vi "Lab Panel V5.28.vi"() -> ()   [LabVIEW 2013] (continued)
                            n1469 = local write "DISP LAB04-1"(w2755) -> ()
                          }
                        }
                      }
                      frame False {
                      }
                    }
                  }
                }
              }
              frame #7 {
                # "LAB04-2"
                n1470 = Equal?(x=w2758, y=2) -> (x = y?=w2761:bool)
                n1471 = local read "DISP LAB04-2"() -> (w2763:T4)
                n1472 = Unbundle(w2763) -> ("STATUS"=w2764:string)  [unwired: 2 out]
                n1473 = Equal?(x=w2764, y="RUN") -> (x = y?=w2760:bool)
                n1474 = And(x=w2760, y=w2761) -> (x .and. y?=w2759:bool)
                n1475 = case shown="True" w2759 {
                  tunnel: w2763 -> [_ w2767]
                  tunnel: w2757 -> [_ w2770]
                  frame False {
                  }
                  frame True {
                    n1476 = local read "SET LAB04-2"() -> (w2769:T5)
                    n1477 = local read "TDMS LAB04-2"() -> (w2766:refnum<k34>)
                    n1478 = Unbundle(w2767) -> ("CYCLE"=w2771:dbl)  [unwired: 2 out]
                    n1479 = Unbundle(w2769) -> ("T-RISE mins"=w2768:dbl)  [unwired: 4 out]
                    n1480 = Greater Or Equal?(x=w2771, y=w2770) -> (x >= y?=w2772:bool)
                    n1481 = case shown="True" w2772 {
                      tunnel: w2768 -> [w2775 _]
                      tunnel: w2767 -> [w2774 _]
                      tunnel: w2766 -> [w2773 _]
                      frame True {
                        n1482 = stacked-sequence {
                          tunnel: w2775 -> [w2778 _]
                          tunnel: w2774 -> [_ w2783]
                          tunnel: w2773 -> [w2776 _]
                          frame #0 {
                            n1483 = Build Array("T-RISE") -> (w2780:string[])
                            n1484 = Build Array(w2778) -> (w2779:dbl[])
                            n1485 = TDMS Write(0:w2776, 5:"TEST PASS", 7:w2780, 9:w2779) -> (15:w2782:errorcluster)  [unwired: 2 in, 3 out]
                            n1486 = local write "data file error"(w2782) -> ()
                          }
                          frame #1 {
                            n1487 = Bundle(cluster=w2783, "STATUS"="T-RISE PASS") -> (w2785:T4)  [unwired: 2 in]
                            n1488 = local write "RESULT LAB04-2"(TRUE) -> ()
                            n1489 = local write "DISP LAB04-2"(w2785) -> ()
                          }
                        }
                      }
                      frame False {
                      }
                    }
                  }
                }
              }
              frame #8 {
                # "LAB05-1"
                n1490 = Equal?(x=w2788, y=2) -> (x = y?=w2791:bool)
                n1491 = local read "DISP LAB05-1"() -> (w2793:T4)
                n1492 = Unbundle(w2793) -> ("STATUS"=w2794:string)  [unwired: 2 out]
                n1493 = Equal?(x=w2794, y="RUN") -> (x = y?=w2790:bool)
                n1494 = And(x=w2790, y=w2791) -> (x .and. y?=w2789:bool)
                n1495 = case shown="True" w2789 {
                  tunnel: w2793 -> [_ w2797]
                  tunnel: w2787 -> [_ w2800]
                  frame False {
                  }
                  frame True {
                    n1496 = local read "SET LAB05-1"() -> (w2799:T5)
                    n1497 = local read "TDMS LAB05-1"() -> (w2796:refnum<k34>)
                    n1498 = Unbundle(w2797) -> ("CYCLE"=w2801:dbl)  [unwired: 2 out]
                    n1499 = Unbundle(w2799) -> ("T-RISE mins"=w2798:dbl)  [unwired: 4 out]
                    n1500 = Greater Or Equal?(x=w2801, y=w2800) -> (x >= y?=w2802:bool)
                    n1501 = case shown="True" w2802 {
                      tunnel: w2798 -> [w2805 _]
                      tunnel: w2797 -> [w2804 _]
                      tunnel: w2796 -> [w2803 _]
                      frame True {
                        n1502 = stacked-sequence {
                          tunnel: w2805 -> [w2808 _]
                          tunnel: w2804 -> [_ w2813]
                          tunnel: w2803 -> [w2806 _]
                          frame #0 {
                            n1503 = Build Array("T-RISE") -> (w2810:string[])
                            n1504 = Build Array(w2808) -> (w2809:dbl[])
                            n1505 = TDMS Write(0:w2806, 5:"TEST PASS", 7:w2810, 9:w2809) -> (15:w2812:errorcluster)  [unwired: 2 in, 3 out]
                            n1506 = local write "data file error"(w2812) -> ()
                          }
                          frame #1 {
                            n1507 = Bundle(cluster=w2813, "STATUS"="T-RISE PASS") -> (w2815:T4)  [unwired: 2 in]
                            n1508 = local write "RESULT LAB05-1"(TRUE) -> ()
                            n1509 = local write "DISP LAB05-1"(w2815) -> ()
                          }
                        }
                      }
                      frame False {
                      }
                    }
                  }
                }
              }
              frame #9 {
                # "LAB05-2"
                n1510 = Equal?(x=w2818, y=2) -> (x = y?=w2821:bool)
                n1511 = local read "DISP LAB05-2"() -> (w2823:T4)
                n1512 = Unbundle(w2823) -> ("STATUS"=w2824:string)  [unwired: 2 out]
                n1513 = Equal?(x=w2824, y="RUN") -> (x = y?=w2820:bool)
                n1514 = And(x=w2820, y=w2821) -> (x .and. y?=w2819:bool)
                n1515 = case shown="True" w2819 {
                  tunnel: w2823 -> [_ w2827]
                  tunnel: w2817 -> [_ w2830]
                  frame False {
                  }
                  frame True {
                    n1516 = local read "SET LAB05-2"() -> (w2829:T5)
                    n1517 = local read "TDMS LAB05-2"() -> (w2826:refnum<k34>)
                    n1518 = Unbundle(w2827) -> ("CYCLE"=w2831:dbl)  [unwired: 2 out]
                    n1519 = Unbundle(w2829) -> ("T-RISE mins"=w2828:dbl)  [unwired: 4 out]
                    n1520 = Greater Or Equal?(x=w2831, y=w2830) -> (x >= y?=w2832:bool)
                    n1521 = case shown="True" w2832 {
                      tunnel: w2828 -> [w2835 _]
                      tunnel: w2827 -> [w2834 _]
                      tunnel: w2826 -> [w2833 _]
                      frame True {
                        n1522 = stacked-sequence {
                          tunnel: w2835 -> [w2838 _]
                          tunnel: w2834 -> [_ w2843]
                          tunnel: w2833 -> [w2836 _]
                          frame #0 {
                            n1523 = Build Array("T-RISE") -> (w2840:string[])
                            n1524 = Build Array(w2838) -> (w2839:dbl[])
                            n1525 = TDMS Write(0:w2836, 5:"TEST PASS", 7:w2840, 9:w2839) -> (15:w2842:errorcluster)  [unwired: 2 in, 3 out]
                            n1526 = local write "data file error"(w2842) -> ()
                          }
                          frame #1 {
                            n1527 = Bundle(cluster=w2843, "STATUS"="T-RISE PASS") -> (w2845:T4)  [unwired: 2 in]
                            n1528 = local write "RESULT LAB05-2"(TRUE) -> ()
                            n1529 = local write "DISP LAB05-2"(w2845) -> ()
                          }
                        }
                      }
                      frame False {
                      }
                    }
                  }
                }
              }
            }
          }
          frame #7 {
            # "end test & close test files"
            n1530 = local read "MAIL SETTINGS"() -> (w2852:T7)
            n1531 = local read "TO (string):"() -> (w2847:string)
            n1532 = Unbundle(w2852) -> ("OUT SERVER ADDRESS"=w2851:string, "FROM ACCOUNT"=w2850:string)  [unwired: 5 out]
            n1533 = stacked-sequence {
              tunnel: w2862 -> [_ _ _ _ _ _ _ _ _ _]
              tunnel: w2863 -> [_ _ _ _ _ _ _ _ _ _]
              tunnel: w2861 -> [_ _ _ _ _ _ _ _ _ _]
              tunnel: w2860 -> [_ _ _ _ _ _ _ _ _ _]
              tunnel: w2859 -> [_ _ _ _ _ _ _ _ _ _]
              tunnel: w2858 -> [_ _ _ _ _ _ _ _ _ _]
              tunnel: w2857 -> [_ _ _ _ _ _ _ _ _ _]
              tunnel: w2856 -> [_ _ _ _ _ _ _ _ _ _]
              tunnel: w2855 -> [_ _ _ _ _ _ _ _ _ _]
              tunnel: w2854 -> [_ _ _ _ _ _ _ _ _ _]
              tunnel: w2851 -> [w2868 w2919 w2967 w3014 w3061 w3108 w3155 w3202 w3249 w3296]
              tunnel: w2850 -> [w2867 w2918 w2966 w3013 w3060 w3107 w3154 w3201 w3248 w3295]
              tunnel: "Mail Test File To:" -> [w2866 w2917 w2965 w3012 w3059 w3106 w3153 w3200 w3247 w3294]
              tunnel: "Mail Test Fail" -> [w2865 w2916 w2964 w3011 w3058 w3105 w3152 w3199 w3246 w3293]
              frame #0 {
                # "LAB01-1"
                n1534 = local read "DISP LAB01-1"() -> (w2864:T4)
                n1535 = global write "Global display 2.vi" "DISP LAB01-1"(w2864) -> ()
                n1536 = local read "run lab01-1"() -> (w2869:bool)
                n1537 = local read "TDMS LAB01-1"() -> (w2870:refnum<k34>)
                n1538 = Unbundle(w2864) -> ("CYCLE"=w2872:dbl, "STATUS"=w2871:string)  [unwired: 1 out]
                n1539 = case shown="True" w2869 {
                  tunnel: w2872 -> [_ w2878]
                  tunnel: w2864 -> [_ w2880]
                  tunnel: w2871 -> [_ w2877]
                  tunnel: w2870 -> [_ w2879]
                  tunnel: w2868 -> [_ w2876]
                  tunnel: w2867 -> [_ w2875]
                  tunnel: w2866 -> [_ w2874]
                  tunnel: w2865 -> [_ w2873]
                  frame False {
                  }
                  frame True {
                    n1540 = Not Equal?(x=w2877, y="RUN") -> (x != y?=w2881:bool)
                    n1541 = Greater?(x=w2878, y=2.0) -> (0:w2883:bool)
                    n1542 = And(x=w2883, y=w2881) -> (x .and. y?=w2882:bool)
                    n1543 = case shown="True" w2882 {
                      tunnel: w2880 -> [_ w2893]
                      tunnel: w2879 -> [_ w2892]
                      tunnel: w2878 -> [_ w2891]
                      tunnel: w2877 -> [_ w2890]
                      tunnel: w2876 -> [_ w2889]
                      tunnel: w2875 -> [_ w2888]
                      tunnel: w2874 -> [_ w2887]
                      tunnel: w2873 -> [_ w2886]
                      frame False {
                      }
                      frame True {
                        n1544 = stacked-sequence {
                          tunnel: w2893 -> [w2897 _ _]
                          tunnel: w2892 -> [_ w2899 _]
                          tunnel: w2891 -> [_ _ _]
                          tunnel: w2890 -> [_ _ w2905]
                          tunnel: w2889 -> [_ _ w2904]
                          tunnel: w2888 -> [_ _ w2903]
                          tunnel: w2887 -> [_ _ w2902]
                          tunnel: w2886 -> [_ _ w2901]
                          frame #0 {
                            w2894 = FALSE
                            n1545 = local write "mail control"("END") -> ()
                            n1546 = Bundle(cluster=w2897) -> (w2896:T4)  [unwired: 3 in]
                            n1547 = local write "DISP LAB01-1"(w2896) -> ()
                            n1548 = local write "O/I  LAB01-1"(w2894) -> ()
                            n1549 = local write "run lab01-1"(w2894) -> ()
                            n1550 = local write "RUN LAB01-1"(w2894) -> ()
                          }
                          frame #1 {
                            n1551 = TDMS Close(11:w2899) -> (0:w2898:errorcluster)  [unwired: 1 in, 1 out]
                            n1552 = local write "data file error"(w2898) -> ()
                          }
                          frame #2 {
                            n1553 = stacked-sequence {
                              tunnel: "LAB01-1" -> [w2907 w2909 _]
                              tunnel: w2905 -> [_ w2915 _]
                              tunnel: w2904 -> [_ w2914 _]
                              tunnel: w2903 -> [_ w2913 _]
                              tunnel: w2902 -> [_ w2912 _]
                              tunnel: w2901 -> [_ w2911 _]
                              frame #0 {
                                n1554 = call "sub vi - defrag tdms v1.vi"("panel id"=w2907) -> ("error out"=w2906:errorcluster)  [unwired: 10 in]
                                n1555 = local write "data file error"(w2906) -> ()
                              }
                              frame #1 {
                                n1556 = Bundle("STATUS"=w2915, "OUT SERVER ADDRESS"=w2914, "FROM ACCOUNT"=w2913, "Mail Test File To:"=w2912, "Mail Test Fail"=w2911) -> (w2908:T26)  [unwired: 1 in]
                                n1557 = call "Save data file (pass-fail) v5.vi"("Input Cluster"=w2908, "panel id"=w2909) -> ("network file save error"=w2910:errorcluster)  [unwired: 8 in, 1 out]
                                n1558 = local write "data file error"(w2910) -> ()
                              }
                              frame #2 {
                              }
                            }
                          }
                        }
                      }
                    }
                  }
                }
              }
              frame #1 {
                # "LAB01-2"
                n1559 = local read "run lab01-2"() -> (w2920:bool)
                n1560 = case shown="True" w2920 {
                  tunnel: w2919 -> [_ w2925]
                  tunnel: w2918 -> [_ w2924]
                  tunnel: w2917 -> [_ w2923]
                  tunnel: w2916 -> [_ w2922]
                  frame False {
                  }
                  frame True {
                    n1561 = local read "DISP LAB01-2"() -> (w2921:T4)
                    n1562 = global write "Global display 2.vi" "DISP LAB01-2"(w2921) -> ()
                    n1563 = local read "TDMS LAB01-2"() -> (w2932:refnum<k34>)
                    n1564 = Unbundle(w2921) -> ("CYCLE"=w2927:dbl, "STATUS"=w2926:string)  [unwired: 1 out]
                    n1565 = Not Equal?(x=w2926, y="RUN") -> (x != y?=w2929:bool)
                    n1566 = Greater?(x=w2927, y=2.0) -> (0:w2930:bool)
                    n1567 = And(x=w2930, y=w2929) -> (x .and. y?=w2928:bool)
                    n1568 = case shown="True" w2928 {
                      tunnel: w2921 -> [_ w2941]
                      tunnel: w2932 -> [_ w2940]
                      tunnel: w2927 -> [_ w2939]
                      tunnel: w2926 -> [_ w2938]
                      tunnel: w2925 -> [_ w2937]
                      tunnel: w2924 -> [_ w2936]
                      tunnel: w2923 -> [_ w2935]
                      tunnel: w2922 -> [_ w2934]
                      frame False {
                      }
                      frame True {
                        n1569 = stacked-sequence {
                          tunnel: w2941 -> [w2944 _ _]
                          tunnel: w2940 -> [_ w2946 _]
                          tunnel: w2939 -> [_ _ _]
                          tunnel: w2938 -> [_ _ w2952]
                          tunnel: w2937 -> [_ _ w2951]
                          tunnel: w2936 -> [_ _ w2950]
                          tunnel: w2935 -> [_ _ w2949]
                          tunnel: w2934 -> [_ _ w2948]
                          frame #0 {
                            w2942 = FALSE
                            n1570 = local write "mail control"("END") -> ()
                            n1571 = Bundle(cluster=w2944) -> (w2945:T4)  [unwired: 3 in]
                            n1572 = local write "RUN LAB01-2"(w2942) -> ()
                            n1573 = local write "run lab01-2"(w2942) -> ()
                            n1574 = local write "O/I  LAB01-2"(w2942) -> ()
                            n1575 = local write "DISP LAB01-2"(w2945) -> ()
                          }
                          frame #1 {
                            n1576 = TDMS Close(11:w2946) -> (0:w2947:errorcluster)  [unwired: 1 in, 1 out]
                            n1577 = local write "data file error"(w2947) -> ()
                          }
                          frame #2 {
                            n1578 = stacked-sequence {
                              tunnel: "LAB01-2" -> [w2955 w2956]
                              tunnel: w2952 -> [_ w2961]
                              tunnel: w2951 -> [_ w2960]
                              tunnel: w2950 -> [_ w2959]
                              tunnel: w2949 -> [_ w2958]
                              tunnel: w2948 -> [_ w2957]
                              frame #0 {
                                n1579 = call "sub vi - defrag tdms v1.vi"("panel id"=w2955) -> ("error out"=w2954:errorcluster)  [unwired: 10 in]
                                n1580 = local write "data file error"(w2954) -> ()
                              }
                              frame #1 {
                                n1581 = Bundle("STATUS"=w2961, "OUT SERVER ADDRESS"=w2960, "FROM ACCOUNT"=w2959, "Mail Test File To:"=w2958, "Mail Test Fail"=w2957) -> (w2963:T26)  [unwired: 1 in]
                                n1582 = call "Save data file (pass-fail) v5.vi"("Input Cluster"=w2963, "panel id"=w2956) -> ("network file save error"=w2962:errorcluster)  [unwired: 8 in, 1 out]
                                n1583 = local write "data file error"(w2962) -> ()
                              }
                            }
                          }
                        }
                      }
                    }
                  }
                }
              }
              frame #2 {
                # "LAB02-1"
                n1584 = local read "run lab02-1"() -> (w2968:bool)
                n1585 = case shown="True" w2968 {
                  tunnel: w2967 -> [_ w2973]
                  tunnel: w2966 -> [_ w2972]
                  tunnel: w2965 -> [_ w2971]
                  tunnel: w2964 -> [_ w2970]
                  frame False {
                  }
                  frame True {
                    n1586 = local read "DISP LAB02-1"() -> (w2969:T4)
                    n1587 = global write "Global display 2.vi" "DISP LAB02-1"(w2969) -> ()
                    n1588 = Unbundle(w2969) -> ("CYCLE"=w2977:dbl, "STATUS"=w2974:string)  [unwired: 1 out]
                    n1589 = local read "TDMS LAB02-1"() -> (w2980:refnum<k34>)
                    n1590 = Not Equal?(x=w2974, y="RUN") -> (x != y?=w2976:bool)
                    n1591 = Greater?(x=w2977, y=2.0) -> (0:w2978:bool)
                    n1592 = And(x=w2978, y=w2976) -> (x .and. y?=w2975:bool)
                    n1593 = case shown="True" w2975 {
                      tunnel: w2969 -> [_ w2988]
                      tunnel: w2980 -> [_ w2987]
                      tunnel: w2974 -> [_ w2986]
                      tunnel: w2973 -> [_ w2985]
                      tunnel: w2972 -> [_ w2984]
                      tunnel: w2971 -> [_ w2983]
                      tunnel: w2970 -> [_ w2982]
                      frame False {
                      }
                      frame True {
                        n1594 = stacked-sequence {
                          tunnel: w2988 -> [w2991 _ _]
                          tunnel: w2987 -> [_ w2993 _]
                          tunnel: w2986 -> [_ _ w2999]
                          tunnel: w2985 -> [_ _ w2998]
                          tunnel: w2984 -> [_ _ w2997]
                          tunnel: w2983 -> [_ _ w2996]
                          tunnel: w2982 -> [_ _ w2995]
                          frame #0 {
                            w2989 = FALSE
                            n1595 = local write "mail control"("END") -> ()
                            n1596 = Bundle(cluster=w2991) -> (w2992:T4)  [unwired: 3 in]
                            n1597 = local write "O/I  LAB02-1"(w2989) -> ()
                            n1598 = local write "RUN LAB02-1"(w2989) -> ()
                            n1599 = local write "run lab02-1"(w2989) -> ()
                            n1600 = local write "DISP LAB02-1"(w2992) -> ()
                          }
                          frame #1 {
                            n1601 = TDMS Close(11:w2993) -> (0:w2994:errorcluster)  [unwired: 1 in, 1 out]
                            n1602 = local write "data file error"(w2994) -> ()
                          }
                          frame #2 {
                            n1603 = stacked-sequence {
                              tunnel: "LAB02-1" -> [w3002 w3009]
                              tunnel: w2999 -> [_ w3007]
                              tunnel: w2998 -> [_ w3006]
                              tunnel: w2997 -> [_ w3005]
                              tunnel: w2996 -> [_ w3004]
                              tunnel: w2995 -> [_ w3003]
                              frame #0 {
                                n1604 = call "sub vi - defrag tdms v1.vi"("panel id"=w3002) -> ("error out"=w3001:errorcluster)  [unwired: 10 in]
                                n1605 = local write "data file error"(w3001) -> ()
                              }
                              frame #1 {
                                n1606 = Bundle("STATUS"=w3007, "OUT SERVER ADDRESS"=w3006, "FROM ACCOUNT"=w3005, "Mail Test File To:"=w3004, "Mail Test Fail"=w3003) -> (w3008:T26)  [unwired: 1 in]
                                n1607 = call "Save data file (pass-fail) v5.vi"("Input Cluster"=w3008, "panel id"=w3009) -> ("network file save error"=w3010:errorcluster)  [unwired: 8 in, 1 out]
                                n1608 = local write "data file error"(w3010) -> ()
                              }
                            }
                          }
                        }
                      }
                    }
                  }
                }
              }
              frame #3 {
                # "LAB02-2"
                n1609 = local read "run lab02-2"() -> (w3015:bool)
                n1610 = case shown="True" w3015 {
                  tunnel: w3014 -> [_ w3021]
                  tunnel: w3013 -> [_ w3020]
                  tunnel: w3012 -> [_ w3019]
                  tunnel: w3011 -> [_ w3018]
                  frame False {
                  }
                  frame True {
                    n1611 = local read "DISP LAB02-2"() -> (w3017:T4)
                    n1612 = global write "Global display 2.vi" "DISP LAB02-2"(w3017) -> ()
                    n1613 = local read "TDMS LAB02-2"() -> (w3027:refnum<k34>)
                    n1614 = Unbundle(w3017) -> ("CYCLE"=w3016:dbl, "STATUS"=w3022:string)  [unwired: 1 out]
                    n1615 = Not Equal?(x=w3022, y="RUN") -> (x != y?=w3024:bool)
                    n1616 = Greater?(x=w3016, y=2.0) -> (0:w3025:bool)
                    n1617 = And(x=w3025, y=w3024) -> (x .and. y?=w3023:bool)
                    n1618 = case shown="True" w3023 {
                      tunnel: w3017 -> [_ w3035]
                      tunnel: w3027 -> [_ w3034]
                      tunnel: w3022 -> [_ w3033]
                      tunnel: w3021 -> [_ w3032]
                      tunnel: w3020 -> [_ w3031]
                      tunnel: w3019 -> [_ w3030]
                      tunnel: w3018 -> [_ w3029]
                      frame False {
                      }
                      frame True {
                        n1619 = stacked-sequence {
                          tunnel: w3035 -> [w3038 _ _]
                          tunnel: w3034 -> [_ w3040 _]
                          tunnel: w3033 -> [_ _ w3046]
                          tunnel: w3032 -> [_ _ w3045]
                          tunnel: w3031 -> [_ _ w3044]
                          tunnel: w3030 -> [_ _ w3043]
                          tunnel: w3029 -> [_ _ w3042]
                          frame #0 {
                            w3036 = FALSE
                            n1620 = local write "mail control"("END") -> ()
                            n1621 = Bundle(cluster=w3038) -> (w3039:T4)  [unwired: 3 in]
                            n1622 = local write "O/I  LAB02-2"(w3036) -> ()
                            n1623 = local write "run lab02-2"(w3036) -> ()
                            n1624 = local write "RUN LAB02-2"(w3036) -> ()
                            n1625 = local write "DISP LAB02-2"(w3039) -> ()
                          }
                          frame #1 {
                            n1626 = TDMS Close(11:w3040) -> (0:w3041:errorcluster)  [unwired: 1 in, 1 out]
                            n1627 = local write "data file error"(w3041) -> ()
                          }
                          frame #2 {
                            n1628 = stacked-sequence {
                              tunnel: "LAB02-2" -> [w3049 w3055]
                              tunnel: w3046 -> [_ w3054]
                              tunnel: w3045 -> [_ w3053]
                              tunnel: w3044 -> [_ w3052]
                              tunnel: w3043 -> [_ w3051]
                              tunnel: w3042 -> [_ w3050]
                              frame #0 {
                                n1629 = call "sub vi - defrag tdms v1.vi"("panel id"=w3049) -> ("error out"=w3048:errorcluster)  [unwired: 10 in]
                                n1630 = local write "data file error"(w3048) -> ()
                              }
                              frame #1 {
                                n1631 = Bundle("STATUS"=w3054, "OUT SERVER ADDRESS"=w3053, "FROM ACCOUNT"=w3052, "Mail Test File To:"=w3051, "Mail Test Fail"=w3050) -> (w3057:T26)  [unwired: 1 in]
                                n1632 = call "Save data file (pass-fail) v5.vi"("Input Cluster"=w3057, "panel id"=w3055) -> ("network file save error"=w3056:errorcluster)  [unwired: 8 in, 1 out]
                                n1633 = local write "data file error"(w3056) -> ()
                              }
                            }
                          }
                        }
                      }
                    }
                  }
                }
              }
              frame #4 {
                # "LAB03-1"
                n1634 = local read "run lab03-1"() -> (w3062:bool)
                n1635 = case shown="True" w3062 {
                  tunnel: w3061 -> [_ w3067]
                  tunnel: w3060 -> [_ w3066]
                  tunnel: w3059 -> [_ w3065]
                  tunnel: w3058 -> [_ w3064]
                  frame False {
                  }
                  frame True {
                    n1636 = local read "DISP LAB03-1"() -> (w3063:T4)
                    n1637 = local read "TDMS LAB03-1"() -> (w3074:refnum<k34>)
                    n1638 = global write "Global display 2.vi" "DISP LAB03-1"(w3063) -> ()
                    n1639 = Unbundle(w3063) -> ("CYCLE"=w3071:dbl, "STATUS"=w3068:string)  [unwired: 1 out]
                    n1640 = Not Equal?(x=w3068, y="RUN") -> (x != y?=w3070:bool)
                    n1641 = Greater?(x=w3071, y=2.0) -> (0:w3072:bool)
                    n1642 = And(x=w3072, y=w3070) -> (x .and. y?=w3069:bool)
                    n1643 = case shown="True" w3069 {
                      tunnel: w3063 -> [_ w3082]
                      tunnel: w3074 -> [_ w3081]
                      tunnel: w3068 -> [_ w3080]
                      tunnel: w3067 -> [_ w3079]
                      tunnel: w3066 -> [_ w3078]
                      tunnel: w3065 -> [_ w3077]
                      tunnel: w3064 -> [_ w3076]
                      frame False {
                      }
                      frame True {
                        n1644 = stacked-sequence {
                          tunnel: w3082 -> [w3085 _ _]
                          tunnel: w3081 -> [_ w3087 _]
                          tunnel: w3080 -> [_ _ w3093]
                          tunnel: w3079 -> [_ _ w3092]
                          tunnel: w3078 -> [_ _ w3091]
                          tunnel: w3077 -> [_ _ w3090]
                          tunnel: w3076 -> [_ _ w3089]
                          frame #0 {
                            w3083 = FALSE
                            n1645 = local write "mail control"("END") -> ()
                            n1646 = Bundle(cluster=w3085) -> (w3086:T4)  [unwired: 3 in]
                            n1647 = local write "O/I  LAB03-1"(w3083) -> ()
                            n1648 = local write "run lab03-1"(w3083) -> ()
                            n1649 = local write "RUN LAB03-1"(w3083) -> ()
                            n1650 = local write "DISP LAB03-1"(w3086) -> ()
                          }
                          frame #1 {
                            n1651 = TDMS Close(11:w3087) -> (0:w3088:errorcluster)  [unwired: 1 in, 1 out]
                            n1652 = local write "data file error"(w3088) -> ()
                          }
                          frame #2 {
                            n1653 = stacked-sequence {
                              tunnel: "LAB03-1" -> [w3096 w3102]
                              tunnel: w3093 -> [_ w3101]
                              tunnel: w3092 -> [_ w3100]
                              tunnel: w3091 -> [_ w3099]
                              tunnel: w3090 -> [_ w3098]
                              tunnel: w3089 -> [_ w3097]
                              frame #0 {
                                n1654 = call "sub vi - defrag tdms v1.vi"("panel id"=w3096) -> ("error out"=w3095:errorcluster)  [unwired: 10 in]
                                n1655 = local write "data file error"(w3095) -> ()
                              }
                              frame #1 {
                                n1656 = Bundle("STATUS"=w3101, "OUT SERVER ADDRESS"=w3100, "FROM ACCOUNT"=w3099, "Mail Test File To:"=w3098, "Mail Test Fail"=w3097) -> (w3104:T26)  [unwired: 1 in]
                                n1657 = call "Save data file (pass-fail) v5.vi"("Input Cluster"=w3104, "panel id"=w3102) -> ("network file save error"=w3103:errorcluster)  [unwired: 8 in, 1 out]
                                n1658 = local write "data file error"(w3103) -> ()
                              }
                            }
                          }
                        }
                      }
                    }
                  }
                }
              }
              frame #5 {
                # "LAB03-2"
                n1659 = local read "run lab03-2"() -> (w3109:bool)
                n1660 = case shown="True" w3109 {
                  tunnel: w3108 -> [_ w3114]
                  tunnel: w3107 -> [_ w3113]
                  tunnel: w3106 -> [_ w3112]
                  tunnel: w3105 -> [_ w3111]
                  frame False {
                  }
                  frame True {
                    n1661 = local read "DISP LAB03-2"() -> (w3110:T4)
                    n1662 = global write "Global display 2.vi" "DISP LAB03-2"(w3110) -> ()
                    n1663 = Unbundle(w3110) -> ("CYCLE"=w3118:dbl, "STATUS"=w3115:string)  [unwired: 1 out]
                    n1664 = local read "TDMS LAB03-2"() -> (w3121:refnum<k34>)
                    n1665 = Not Equal?(x=w3115, y="RUN") -> (x != y?=w3117:bool)
                    n1666 = Greater?(x=w3118, y=2.0) -> (0:w3119:bool)
                    n1667 = And(x=w3119, y=w3117) -> (x .and. y?=w3116:bool)
                    n1668 = case shown="True" w3116 {
                      tunnel: w3110 -> [_ w3129]
                      tunnel: w3121 -> [_ w3128]
                      tunnel: w3115 -> [_ w3127]
                      tunnel: w3114 -> [_ w3126]
                      tunnel: w3113 -> [_ w3125]
                      tunnel: w3112 -> [_ w3124]
                      tunnel: w3111 -> [_ w3123]
                      frame False {
                      }
                      frame True {
                        n1669 = stacked-sequence {
                          tunnel: w3129 -> [w3132 _ _]
                          tunnel: w3128 -> [_ w3134 _]
                          tunnel: w3127 -> [_ _ w3140]
                          tunnel: w3126 -> [_ _ w3139]
                          tunnel: w3125 -> [_ _ w3138]
                          tunnel: w3124 -> [_ _ w3137]
                          tunnel: w3123 -> [_ _ w3136]
                          frame #0 {
                            w3130 = FALSE
                            n1670 = local write "mail control"("END") -> ()
                            n1671 = Bundle(cluster=w3132) -> (w3133:T4)  [unwired: 3 in]
                            n1672 = local write "RUN LAB03-2"(w3130) -> ()
                            n1673 = local write "O/I  LAB03-2"(w3130) -> ()
                            n1674 = local write "DISP LAB03-2"(w3133) -> ()
                            n1675 = local write "run lab03-2"(w3130) -> ()
                          }
                          frame #1 {
                            n1676 = TDMS Close(11:w3134) -> (0:w3135:errorcluster)  [unwired: 1 in, 1 out]
                            n1677 = local write "data file error"(w3135) -> ()
                          }
                          frame #2 {
                            n1678 = stacked-sequence {
                              tunnel: "LAB03-2" -> [w3143 w3144]
                              tunnel: w3140 -> [_ w3149]
                              tunnel: w3139 -> [_ w3148]
                              tunnel: w3138 -> [_ w3147]
                              tunnel: w3137 -> [_ w3146]
                              tunnel: w3136 -> [_ w3145]
                              frame #0 {
                                n1679 = call "sub vi - defrag tdms v1.vi"("panel id"=w3143) -> ("error out"=w3142:errorcluster)  [unwired: 10 in]
                                n1680 = local write "data file error"(w3142) -> ()
                              }
                              frame #1 {
                                n1681 = Bundle("STATUS"=w3149, "OUT SERVER ADDRESS"=w3148, "FROM ACCOUNT"=w3147, "Mail Test File To:"=w3146, "Mail Test Fail"=w3145) -> (w3151:T26)  [unwired: 1 in]
                                n1682 = call "Save data file (pass-fail) v5.vi"("Input Cluster"=w3151, "panel id"=w3144) -> ("network file save error"=w3150:errorcluster)  [unwired: 8 in, 1 out]
                                n1683 = local write "data file error"(w3150) -> ()
                              }
                            }
                          }
                        }
                      }
                    }
                  }
                }
              }
              frame #6 {
                # "LAB04-1"
                n1684 = local read "run lab04-1"() -> (w3156:bool)
                n1685 = case shown="True" w3156 {
                  tunnel: w3155 -> [_ w3161]
                  tunnel: w3154 -> [_ w3160]
                  tunnel: w3153 -> [_ w3159]
                  tunnel: w3152 -> [_ w3158]
                  frame False {
                  }
                  frame True {
                    n1686 = local read "DISP LAB04-1"() -> (w3157:T4)
                    n1687 = Unbundle(w3157) -> ("CYCLE"=w3165:dbl, "STATUS"=w3162:string)  [unwired: 1 out]
                    n1688 = local read "TDMS LAB04-1"() -> (w3168:refnum<k34>)
                    n1689 = global write "Global display 2.vi" "DISP LAB04-1"(w3157) -> ()
                    n1690 = Not Equal?(x=w3162, y="RUN") -> (x != y?=w3164:bool)
                    n1691 = Greater?(x=w3165, y=2.0) -> (0:w3166:bool)
                    n1692 = And(x=w3166, y=w3164) -> (x .and. y?=w3163:bool)
                    n1693 = case shown="True" w3163 {
                      tunnel: w3157 -> [_ w3176]
                      tunnel: w3168 -> [_ w3175]
                      tunnel: w3162 -> [_ w3174]
                      tunnel: w3161 -> [_ w3173]
                      tunnel: w3160 -> [_ w3172]
                      tunnel: w3159 -> [_ w3171]
                      tunnel: w3158 -> [_ w3170]
                      frame False {
                      }
                      frame True {
                        n1694 = stacked-sequence {
                          tunnel: w3176 -> [w3179 _ _]
                          tunnel: w3175 -> [_ w3181 _]
                          tunnel: w3174 -> [_ _ w3187]
                          tunnel: w3173 -> [_ _ w3186]
                          tunnel: w3172 -> [_ _ w3185]
                          tunnel: w3171 -> [_ _ w3184]
                          tunnel: w3170 -> [_ _ w3183]
                          frame #0 {
                            w3177 = FALSE
                            n1695 = local write "mail control"("END") -> ()
                            n1696 = Bundle(cluster=w3179) -> (w3180:T4)  [unwired: 3 in]
                            n1697 = local write "RUN LAB04-1"(w3177) -> ()
                            n1698 = local write "O/I  LAB04-1"(w3177) -> ()
                            n1699 = local write "run lab04-1"(w3177) -> ()
                            n1700 = local write "DISP LAB04-1"(w3180) -> ()
                          }
                          frame #1 {
                            n1701 = TDMS Close(11:w3181) -> (0:w3182:errorcluster)  [unwired: 1 in, 1 out]
                            n1702 = local write "data file error"(w3182) -> ()
                          }
                          frame #2 {
                            n1703 = stacked-sequence {
                              tunnel: "LAB04-1" -> [w3190 w3191]
                              tunnel: w3187 -> [_ w3196]
                              tunnel: w3186 -> [_ w3195]
                              tunnel: w3185 -> [_ w3194]
                              tunnel: w3184 -> [_ w3193]
                              tunnel: w3183 -> [_ w3192]
                              frame #0 {
                                n1704 = call "sub vi - defrag tdms v1.vi"("panel id"=w3190) -> ("error out"=w3189:errorcluster)  [unwired: 10 in]
                                n1705 = local write "data file error"(w3189) -> ()
                              }
                              frame #1 {
                                n1706 = Bundle("STATUS"=w3196, "OUT SERVER ADDRESS"=w3195, "FROM ACCOUNT"=w3194, "Mail Test File To:"=w3193, "Mail Test Fail"=w3192) -> (w3198:T26)  [unwired: 1 in]
                                n1707 = call "Save data file (pass-fail) v5.vi"("Input Cluster"=w3198, "panel id"=w3191) -> ("network file save error"=w3197:errorcluster)  [unwired: 8 in, 1 out]
                                n1708 = local write "data file error"(w3197) -> ()
                              }
                            }
                          }
                        }
                      }
                    }
                  }
                }
              }
              frame #7 {
                # "LAB04-2"
                n1709 = local read "run lab04-2"() -> (w3203:bool)
                n1710 = case shown="True" w3203 {
                  tunnel: w3202 -> [_ w3208]
                  tunnel: w3201 -> [_ w3207]
                  tunnel: w3200 -> [_ w3206]
                  tunnel: w3199 -> [_ w3205]
                  frame False {
                  }
                  frame True {
                    n1711 = local read "DISP LAB04-2"() -> (w3204:T4)
                    n1712 = Unbundle(w3204) -> ("CYCLE"=w3212:dbl, "STATUS"=w3209:string)  [unwired: 1 out]
                    n1713 = global write "Global display 2.vi" "DISP LAB04-2"(w3204) -> ()
                    n1714 = Not Equal?(x=w3209, y="RUN") -> (x != y?=w3211:bool)
                    n1715 = local read "TDMS LAB04-2"() -> (w3215:refnum<k34>)
                    n1716 = Greater?(x=w3212, y=2.0) -> (0:w3213:bool)
                    n1717 = And(x=w3213, y=w3211) -> (x .and. y?=w3210:bool)
                    n1718 = case shown="True" w3210 {
                      tunnel: w3204 -> [_ w3223]
                      tunnel: w3215 -> [_ w3222]
                      tunnel: w3209 -> [_ w3221]
                      tunnel: w3208 -> [_ w3220]
                      tunnel: w3207 -> [_ w3219]
                      tunnel: w3206 -> [_ w3218]
                      tunnel: w3205 -> [_ w3217]
                      frame False {
                      }
                      frame True {
                        n1719 = stacked-sequence {
                          tunnel: w3223 -> [w3226 _ _]
                          tunnel: w3222 -> [_ w3228 _]
                          tunnel: w3221 -> [_ _ w3234]
                          tunnel: w3220 -> [_ _ w3233]
                          tunnel: w3219 -> [_ _ w3232]
                          tunnel: w3218 -> [_ _ w3231]
                          tunnel: w3217 -> [_ _ w3230]
                          frame #0 {
                            w3224 = FALSE
                            n1720 = local write "mail control"("END") -> ()
                            n1721 = Bundle(cluster=w3226) -> (w3227:T4)  [unwired: 3 in]
                            n1722 = local write "O/I  LAB04-2"(w3224) -> ()
                            n1723 = local write "RUN LAB04-2"(w3224) -> ()
                            n1724 = local write "run lab04-2"(w3224) -> ()
                            n1725 = local write "DISP LAB04-2"(w3227) -> ()
                          }
                          frame #1 {
                            n1726 = TDMS Close(11:w3228) -> (0:w3229:errorcluster)  [unwired: 1 in, 1 out]
                            n1727 = local write "data file error"(w3229) -> ()
                          }
                          frame #2 {
                            n1728 = stacked-sequence {
                              tunnel: "LAB04-2" -> [w3237 w3238]
                              tunnel: w3234 -> [_ w3243]
                              tunnel: w3233 -> [_ w3242]
                              tunnel: w3232 -> [_ w3241]
                              tunnel: w3231 -> [_ w3240]
                              tunnel: w3230 -> [_ w3239]
                              frame #0 {
                                n1729 = call "sub vi - defrag tdms v1.vi"("panel id"=w3237) -> ("error out"=w3236:errorcluster)  [unwired: 10 in]
                                n1730 = local write "data file error"(w3236) -> ()
                              }
                              frame #1 {
                                n1731 = Bundle("STATUS"=w3243, "OUT SERVER ADDRESS"=w3242, "FROM ACCOUNT"=w3241, "Mail Test File To:"=w3240, "Mail Test Fail"=w3239) -> (w3245:T26)  [unwired: 1 in]
                                n1732 = call "Save data file (pass-fail) v5.vi"("Input Cluster"=w3245, "panel id"=w3238) -> ("network file save error"=w3244:errorcluster)  [unwired: 8 in, 1 out]
                                n1733 = local write "data file error"(w3244) -> ()
                              }
                            }
                          }
                        }
                      }
                    }
                  }
                }
              }
              frame #8 {
                # "LAB05-1"
                n1734 = local read "run lab05-1"() -> (w3250:bool)
                n1735 = case shown="True" w3250 {
                  tunnel: w3249 -> [_ w3255]
                  tunnel: w3248 -> [_ w3254]
                  tunnel: w3247 -> [_ w3253]
                  tunnel: w3246 -> [_ w3252]
                  frame False {
                  }
                  frame True {
                    n1736 = local read "DISP LAB05-1"() -> (w3251:T4)
                    n1737 = Unbundle(w3251) -> ("CYCLE"=w3259:dbl, "STATUS"=w3256:string)  [unwired: 1 out]
                    n1738 = global write "Global display 2.vi" "DISP LAB05-1"(w3251) -> ()
                    n1739 = Not Equal?(x=w3256, y="RUN") -> (x != y?=w3258:bool)
                    n1740 = local read "TDMS LAB05-1"() -> (w3262:refnum<k34>)
                    n1741 = Greater?(x=w3259, y=2.0) -> (0:w3260:bool)
                    n1742 = And(x=w3260, y=w3258) -> (x .and. y?=w3257:bool)
                    n1743 = case shown="True" w3257 {
                      tunnel: w3251 -> [_ w3270]
                      tunnel: w3262 -> [_ w3269]
                      tunnel: w3256 -> [_ w3268]
                      tunnel: w3255 -> [_ w3267]
                      tunnel: w3254 -> [_ w3266]
                      tunnel: w3253 -> [_ w3265]
                      tunnel: w3252 -> [_ w3264]
                      frame False {
                      }
                      frame True {
                        n1744 = stacked-sequence {
                          tunnel: w3270 -> [w3273 _ _]
                          tunnel: w3269 -> [_ w3275 _]
                          tunnel: w3268 -> [_ _ w3281]
                          tunnel: w3267 -> [_ _ w3280]
                          tunnel: w3266 -> [_ _ w3279]
                          tunnel: w3265 -> [_ _ w3278]
                          tunnel: w3264 -> [_ _ w3277]
                          frame #0 {
                            w3271 = FALSE
                            n1745 = local write "mail control"("END") -> ()
                            n1746 = Bundle(cluster=w3273) -> (w3274:T4)  [unwired: 3 in]
                            n1747 = local write "O/I  LAB05-1"(w3271) -> ()
                            n1748 = local write "RUN LAB05-1"(w3271) -> ()
                            n1749 = local write "run lab05-1"(w3271) -> ()
                            n1750 = local write "DISP LAB05-1"(w3274) -> ()
                          }
                          frame #1 {
                            n1751 = TDMS Close(11:w3275) -> (0:w3276:errorcluster)  [unwired: 1 in, 1 out]
                            n1752 = local write "data file error"(w3276) -> ()
                          }
                          frame #2 {
                            n1753 = stacked-sequence {
                              tunnel: "LAB05-1" -> [w3284 w3290]
                              tunnel: w3281 -> [_ w3289]
                              tunnel: w3280 -> [_ w3288]
                              tunnel: w3279 -> [_ w3287]
                              tunnel: w3278 -> [_ w3286]
                              tunnel: w3277 -> [_ w3285]
                              frame #0 {
                                n1754 = call "sub vi - defrag tdms v1.vi"("panel id"=w3284) -> ("error out"=w3283:errorcluster)  [unwired: 10 in]
                                n1755 = local write "data file error"(w3283) -> ()
                              }
                              frame #1 {
                                n1756 = Bundle("STATUS"=w3289, "OUT SERVER ADDRESS"=w3288, "FROM ACCOUNT"=w3287, "Mail Test File To:"=w3286, "Mail Test Fail"=w3285) -> (w3292:T26)  [unwired: 1 in]
                                n1757 = call "Save data file (pass-fail) v5.vi"("Input Cluster"=w3292, "panel id"=w3290) -> ("network file save error"=w3291:errorcluster)  [unwired: 8 in, 1 out]
                                n1758 = local write "data file error"(w3291) -> ()
                              }
                            }
                          }
                        }
                      }
                    }
                  }
                }
              }
              frame #9 {
                # "LAB05-2"
                n1759 = local read "run lab05-2"() -> (w3297:bool)
                n1760 = case shown="True" w3297 {
                  tunnel: w3296 -> [_ w3302]
                  tunnel: w3295 -> [_ w3301]
                  tunnel: w3294 -> [_ w3300]
                  tunnel: w3293 -> [_ w3299]
                  frame False {
                  }
                  frame True {
                    n1761 = local read "DISP LAB05-2"() -> (w3298:T4)
                    n1762 = Unbundle(w3298) -> ("CYCLE"=w3306:dbl, "STATUS"=w3303:string)  [unwired: 1 out]
                    n1763 = global write "Global display 2.vi" "DISP LAB05-2"(w3298) -> ()
                    n1764 = Not Equal?(x=w3303, y="RUN") -> (x != y?=w3305:bool)
                    n1765 = local read "TDMS LAB05-2"() -> (w3309:refnum<k34>)
                    n1766 = Greater?(x=w3306, y=2.0) -> (0:w3307:bool)
                    n1767 = And(x=w3307, y=w3305) -> (x .and. y?=w3304:bool)
                    n1768 = case shown="True" w3304 {
                      tunnel: w3298 -> [_ w3317]
                      tunnel: w3309 -> [_ w3316]
                      tunnel: w3303 -> [_ w3315]
                      tunnel: w3302 -> [_ w3314]
                      tunnel: w3301 -> [_ w3313]
                      tunnel: w3300 -> [_ w3312]
                      tunnel: w3299 -> [_ w3311]
                      frame False {
                      }
                      frame True {
                        n1769 = stacked-sequence {
                          tunnel: w3317 -> [w3320 _ _]
                          tunnel: w3316 -> [_ w3322 _]
                          tunnel: w3315 -> [_ _ w3328]
                          tunnel: w3314 -> [_ _ w3327]
                          tunnel: w3313 -> [_ _ w3326]
                          tunnel: w3312 -> [_ _ w3325]
                          tunnel: w3311 -> [_ _ w3324]
                          frame #0 {
                            w3318 = FALSE
                            n1770 = local write "mail control"("END") -> ()
                            n1771 = Bundle(cluster=w3320) -> (w3321:T4)  [unwired: 3 in]
                            n1772 = local write "RUN LAB05-2"(w3318) -> ()
                            n1773 = local write "O/I  LAB05-2"(w3318) -> ()
